vi "mes初始化.vi"(10 "mes":string[][](array[string])) -> ()   [LabVIEW 2020]
uses:
  Global.vi
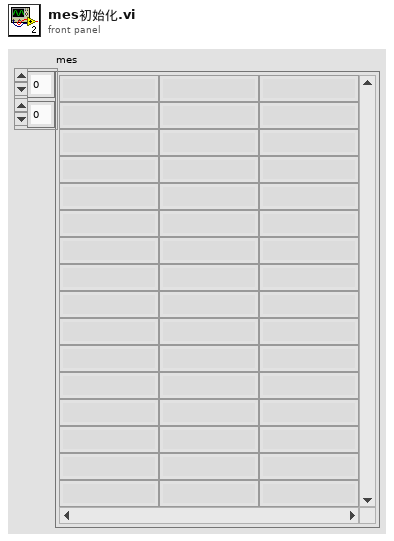
[diagram p1: front panel]
types:
  T1 = cluster{"Server":string, "audit_mode":string, "tsid":string, "model":string, "product":string, "test_station":string, "station_id":string, "test_station_name":string, "Webservice":string}
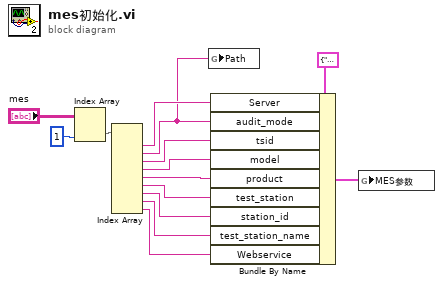
[diagram p0: block diagram]
diagram:
  n1 = Index Array(array="mes", index (col)=1 ("禁用的索引 (列)")) -> (element=w9:string[])  [unwired: 1 in]
  n2 = Index Array(array=w9) -> (element #1=w14:string, element #2=w1:string, element #3=w8:string, element #4=w7:string, element #5=w6:string, element #6=w5:string, element #7=w4:string, element #8=w3:string, element #9=w2:string)  [unwired: 9 in]
  n3 = global write "Global.vi" "Path"(w1) -> ()
  n4 = Bundle By Name(cluster=T1 {"Server"="", "audit_mode"="", "tsid"="", "model"="", "product"="", "test_station"="", "station_id"="", "test_station_name"="", "Webservice"=""} ("MES参数"), "Server"=w14, "audit_mode"=w1, "tsid"=w8, "model"=w7, "product"=w6, "test_station"=w5, "station_id"=w4, "test_station_name"=w3, "Webservice"=w2) -> (w13:T1)
  n5 = global write "Global.vi" "MES参数"(w13) -> ()
